vi "Get Enclave.vi"(8 "error in (no error)":errorcluster, 11 "Event in":refnum<class "Event.lvclass">) -> (0 "error out":errorcluster, 2 "Enclave":refnum<class "Enclave.lvclass">, 3 "Event out":refnum<class "Event.lvclass">)   [LabVIEW 2022 SP3, in "Enclave.lvlib" / "Event.lvclass"]
uses:
  Event.lvclass
  Event.lvclass/Event.ctl
  Enclave/Enclave.lvclass
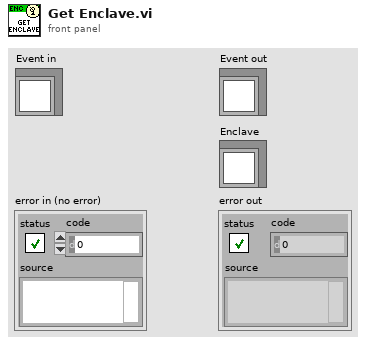
[diagram p1: front panel]
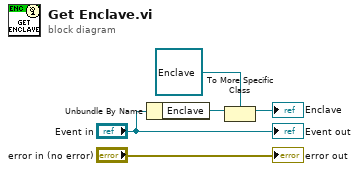
[diagram p0: block diagram]
diagram:
  n1 = Unbundle By Name("Event in") -> ("Enclave"=w4:refnum<class>)
  n2 = To More Specific Class(target class=refnum<class "Enclave.lvclass"> refnum ("Enclave.lvlib:Enclave.lvclass"), reference=w4) -> (specific class reference=→"Enclave":refnum<class "Enclave.lvclass">)  [unwired: 1 in, 1 out]
  "error out" <- "error in (no error)"
  "Event out" <- "Event in"
